vi "Scripting_SortCpControls.vi"(8 "error in (no error)":errorcluster, 11 "Connector Pane:Reference":refnum<vi>) -> (0 "error out":errorcluster, 1 "IndexOnUpperRightCorner":i32, 2 "TermIndex":i32[](array[numeric]), 3 "Controls[]":refnum<vi>[](array[refnum]), 4 "IndexOnLowerRightCorner":i32, 5 "IndexOnUpperLeftCorner":i32, 6 "IndexOnLowerLeftCorner":i32)   [LabVIEW 2014]
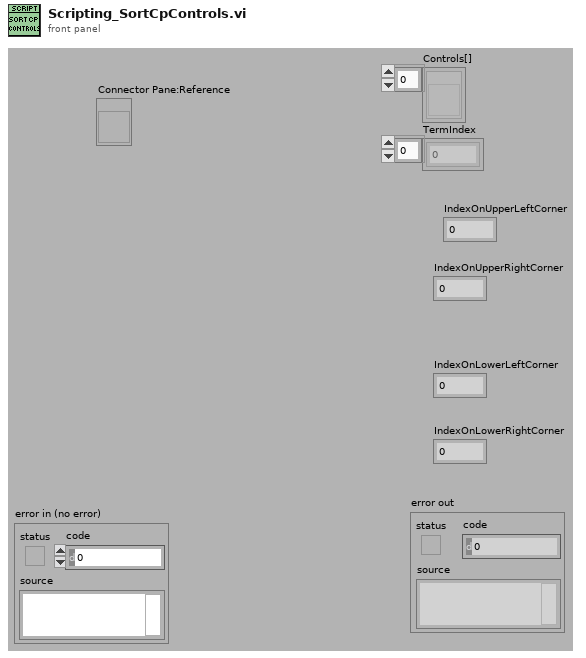
[diagram p1: front panel]
types:
  T1 = typedef "LVRectTypeDef.ctl" = cluster{"Left":i16, "Top":i16, "Right":i16, "Bottom":i16}
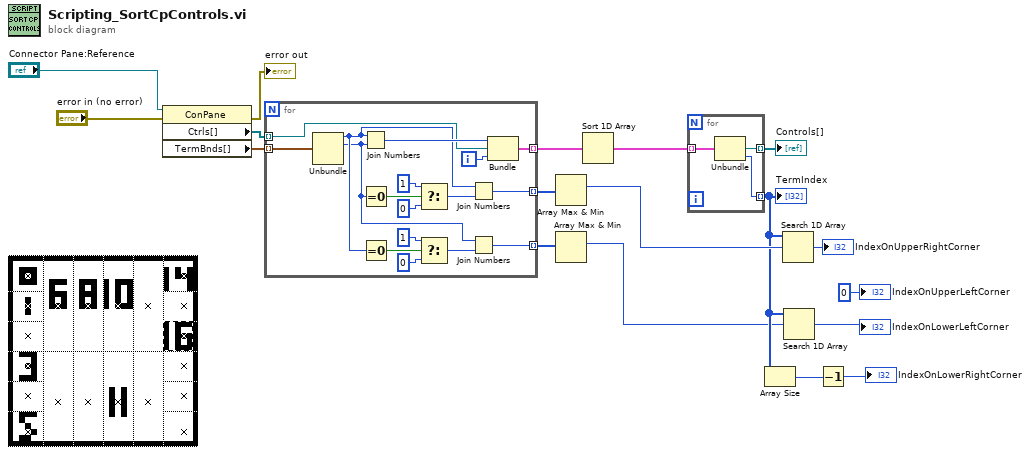
[diagram p0: block diagram]
diagram:
  n1 = property class="ConPane"(reference="Connector Pane:Reference", error in="error in (no error)") -> (error out=→"error out":errorcluster, "Ctrls[]"=w14:refnum<vi>[], "TermBnds[]"=w15:T1[])  [unwired: 1 out]
  n2 = for {
    tunnel: [w34] -> w18 mode=indexing
    tunnel: w15 -> [w33] mode=indexing
    tunnel: w14 -> [w32] mode=indexing
    tunnel: [w26] -> w10 mode=indexing
    tunnel: [w19] -> w4 mode=indexing
    i -> [w31]
    n3 = Unbundle(w33) -> ("Left"=w21:i16, "Top"=w20:i16)  [unwired: 2 out]
    n4 = Join Numbers(hi=w21, lo=w20) -> ((hi.lo)=w35:u32)
    n5 = Equal To 0?(x=w20) -> (x = 0?=w30:bool)
    n6 = Equal To 0?(x=w21) -> (x = 0?=w22:bool)
    n7 = Select(t=i16 1, s=w30, f=i16 0) -> (s? t:f=w29:i16)
    n8 = Select(t=i16 1, s=w22, f=i16 0) -> (s? t:f=w23:i16)
    n9 = Join Numbers(hi=w21, lo=w29) -> ((hi.lo)=w26:u32)
    n10 = Join Numbers(hi=w20, lo=w23) -> ((hi.lo)=w19:u32)
    n11 = Bundle(w35, w32, w31) -> (w34:cluster{u32, refnum<vi>, i32})  [unwired: 1 in]
  }
  n12 = Array Max & Min(array=w10) -> (max index (indices)=w9:i32)  [unwired: 3 out]
  n13 = Array Max & Min(array=w4) -> (max index (indices)=w2:i32)  [unwired: 3 out]
  n14 = Sort 1D Array(array=w18) -> (sorted array=w17:cluster{u32, refnum<vi>, i32}[])
  n15 = for {
    tunnel: w17 -> [w38] mode=indexing
    tunnel: [w37] -> w13 mode=indexing
    tunnel: [w36] -> w3 mode=indexing
    n16 = Unbundle(w38) -> (w37:refnum<vi>, w36:i32)  [unwired: 1 out]
  }
  "Controls[]" <- w13
  "TermIndex" <- w3
  n17 = Array Size(array=w3) -> (size(s)=w7:i32)
  n18 = Search 1D Array(1D array=w3, element=w9) -> (index of element=→"IndexOnUpperRightCorner":i32)  [unwired: 1 in]
  n19 = Search 1D Array(1D array=w3, element=w2) -> (index of element=→"IndexOnLowerLeftCorner":i32)  [unwired: 1 in]
  n20 = Decrement(x=w7) -> (x-1=→"IndexOnLowerRightCorner":i32)
  "IndexOnUpperLeftCorner" <- 0 ("IndexOnUpperLeftCorner")
